vi "Get Session Information.vi"(8 "error in (no error)":errorcluster, 11 "session information":T1[](array[typedef])) -> (0 "error out":errorcluster, 3 "session information":T1)   [LabVIEW 2020, in "NIDCPowerSourceDCVoltage.lvlib"]
uses:
  NIDCPowerSourceDCVoltage.lvlib
  <vilib>/MeasurementLink/MeasurementLink Session Management Client/RPC Messages/ni_measurementlink_sessionmanagement_v1_SessionInformation.ctl
  <vilib>/MeasurementLink/MeasurementLink Session Management Client/RPC Messages/nidevice_grpc_Session.ctl
  <vilib>/MeasurementLink/MeasurementLink Session Management Client/RPC Messages/ni_measurementlink_sessionmanagement_v1_ChannelMapping.ctl
  <vilib>/MeasurementLink/MeasurementLink Session Management Client/MeasurementLink Session Management Client.lvlib
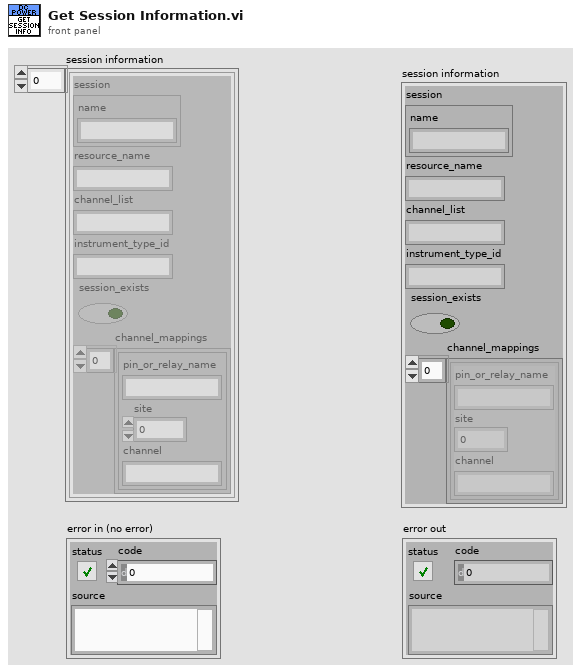
[diagram p1: front panel]
types:
  T1 = typedef "MeasurementLink Session Management Client.lvlib/ni_measurementlink_sessionmanagement_v1_SessionInformation.ctl" = cluster{"session":T2, "resource_name":string, "channel_list":string, "instrument_type_id":string, "session_exists":bool, "channel_mappings":T3[]}
  T2 = typedef "MeasurementLink Session Management Client.lvlib/nidevice_grpc_Session.ctl" = cluster{"name":string}
  T3 = typedef "MeasurementLink Session Management Client.lvlib/ni_measurementlink_sessionmanagement_v1_ChannelMapping.ctl" = cluster{"pin_or_relay_name":string, "site":i32, "channel":string}
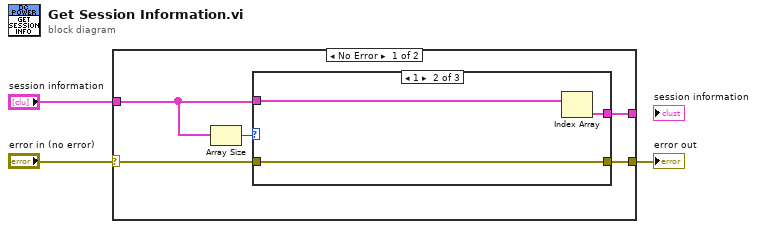
[diagram p0: block diagram]
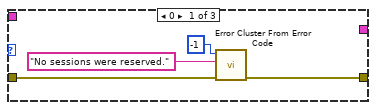
[diagram p2: hidden frame]
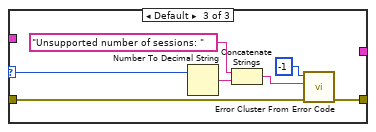
[diagram p3: hidden frame]
diagram:
  n1 = case shown="No Error" "error in (no error)" {
    selector: "error in (no error)" -> [w7 w23]
    tunnel: "session information" -> [w4 _]
    tunnel: [w6 w23] -> w2
    tunnel: [w5 _] -> _
    frame No Error {
      n2 = Array Size(array=w4) -> (size(s)=w8:i32)
      n3 = case shown="1" w8 {
        selector: w8 -> [_ _ w17]
        tunnel: w7 -> [w12 w14 w22]
        tunnel: [w9 w14 w20] -> w6
        tunnel: w4 -> [_ w13 _]
        tunnel: [_ w15 _] -> w5
        frame 0 {
          n4 = call <vilib>:"Error Cluster From Error Code.vi"("error in (no error)"=w12, "error message (\"\")"="No sessions were reserved." ("error message (\"\")"), "error code (0)"=-1) -> ("error out"=w9:errorcluster)  [unwired: 6 in]
        }
        frame 1 {
          n5 = Index Array(array=w13) -> (element=w15:T1)  [unwired: 1 in]
        }
        frame Default {
          n6 = Number To Decimal String(number=w17) -> (decimal integer string=w18:string)  [unwired: 1 in]
          n7 = Concatenate Strings("Unsupported number of sessions: " ("error message (\"\")"), w18) -> (w16:string)
          n8 = call <vilib>:"Error Cluster From Error Code.vi"("error in (no error)"=w22, "error message (\"\")"=w16, "error code (0)"=-1) -> ("error out"=w20:errorcluster)  [unwired: 6 in]
        }
      }
    }
    frame Error {
    }
  }
  "error out" <- w2
